vi "Configure Sequencer List Filling Frequency.vi"(7 "Increment (0.0)":dbl format="%^.3e", 8 "error in (no error)":errorcluster, 9 "Start Value (1.2E+9)":dbl=1200000000.0 format="%^.3e", 10 "Instance (1)":i32=1, 11 "VISA resource name":refnum<visa-resource-name>) -> (0 "error out":errorcluster, 3 "VISA resource name out":refnum<visa-resource-name>)   [LabVIEW 2020, in "Rohde&Schwarz CMXP GPRF.lvlib"]
doc: "Configures the values for filling the sequencer list with frequency values.\n\nAttributes:\nRSCMXPGPRF_ATTR_SEQUENCER_LIST_FILLING_FREQUENCY_START_VALUE\nRSCMXPGPRF_ATTR_SEQUENCER_LIST_FILLING_FREQUENCY_INCREMENT\n\nRemote-control commands:\nSOURce:GPRF:GEN<i>:SEQuencer:LIST:FILL:FREQuency:SVALue\nSOURce:GPRF:GEN<i>:SEQuencer:LIST:FILL:FREQuency:INCRement"
uses:
  <instrlib>/Rohde&Schwarz CMXP GPRF/Rohde&Schwarz CMXP GPRF.lvlib
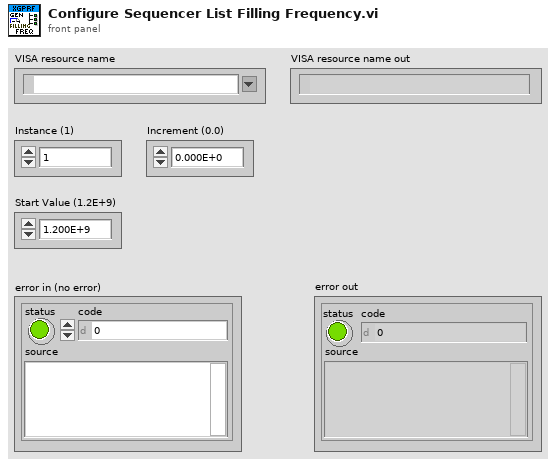
[diagram p1: front panel]
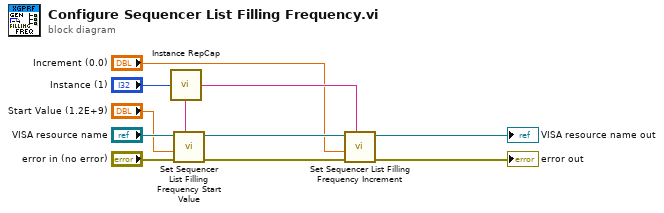
[diagram p0: block diagram]
diagram:
  n1 = call <instrlib>:"Instance RepCap.vi"("Instance in"="Instance (1)") -> ("Instance out"=w3:string)
  n2 = call "Set Sequencer List Filling Frequency Start Value"("Repeated Capabilities"=w3, "error in (no error)"="error in (no error)", "Sequencer List Filling Frequency Start Value (0.0)"="Start Value (1.2E+9)", "instrument handle"="VISA resource name") -> ("error out"=w5:errorcluster, "instrument handle out"=w6:refnum<visa-resource-name>)  [unwired: 6 in]
  n3 = call "Set Sequencer List Filling Frequency Increment"("Repeated Capabilities"=w3, "error in (no error)"=w5, "Sequencer List Filling Frequency Increment (0.0)"="Increment (0.0)", "instrument handle"=w6) -> ("error out"=→"error out":errorcluster, "instrument handle out"=→"VISA resource name out":refnum<visa-resource-name>)  [unwired: 6 in]
